vi "Topo & GridSpectr_DriftCorrection_zSpec_v20.vi"(6 "Internal use":string, 7 "Grid param":T2 {"height (m)" format="%#_6p"; "width (m)" format="%#_6p"; "center Y (m)" format="%#_6p"; "center X (m)" format="%#_6p"}, 8 "Error in (no error)":errorcluster, 9 "Points Y/Index Y":i32, 10 "Points X/Index X":i32, 11 "Method":enum16{"init", "run", "end"}(ring)=enum."end") -> (0 "Error out":errorcluster)   [LabVIEW 2014]
doc: "Example of a measurement VI to be used in the \"Experiments on a Grid\" tool as external VI.\n\nThis example measure the topography and spectroscopy data. The spectroscopy measurements are taken on a subgrid. The data are saved to a sxm and a binary file.\n\n- Nanonis Programming Interface -"
uses:
  <userlib>/Nanonis Prog Interface V5/Nanonis Prog Interface.lvlib
panel:
  out "output cluster":T1
  in  "PLL ON/OFF":bool=TRUE
  in  "Spectroscopy":u16(ring) items=["Bias", "zSpec"]
  in  "autoStop":bool
  in  "trigger 2 >Hz":sgl format="%#_6p"
  in  "trigger1 < Hz":sgl format="%#_6p"
  out "zFile":refnum<file>
  out "last z adjustment":sgl=-8.2707174e-12 format="%#_6p"
  in  "during Spec Bias (V)":sgl=-0.1 format="%#_5p"
  in  "type":u16(ring)=1 items=["Line", "Grid"]
  in  "readjust setpoint every":i32=1
  in  "Correct Drift":bool=TRUE
  in  "Email when finished":string="cornelius.krull@monash.edu,Dhaneesh.Gopalakrishnan@monash.edu,marina.castelli@monash.edu"
  in  "STS z offset":dbl=2e-10 format="%#_6p"
  out "ETA":timestamp=timestamp(3575267058.899443 s since 1904-01-01)
  out "remaining":dbl format="%<%H:%M:%S>t"
  out "Progress":u8(slide)=100 scale=0.0..100.0 scale format="%#.1g"
  out "total Points":i32=2500
  in  "preSTS delay [ms]":u32=500
  in  "ref Bias":dbl=-0.1 format="%#_6p"
  in  "Imaging Bias":dbl=0.02 format="%#_6p"
  in  "max applied Drift Correction":i32=20 min=1 max=100 step=1 format="%.0p"
  in  "Correlate":u16(ring) items=["first Frame", "successive Frames"]
  out "Topo Images taken":i32=50
  in  "Increment":i32=8
  in  "Threshold":i32=2 min=1 step=1
  in  "tip Speed (m/s)":sgl=2e-09 format="%.2p"
  out "X drift":i32=1
  out "Y drift":i32
  out "Last Drift detected":i32=1
  in  "MaxImagesBack":i32=2
  in  "Channel index (0-23)":u8(ring) items=["Current"=0, "Z (m)"=14]
  in  "File name":string="symmetric_node_zOff=200p"
  in  "ref Current":dbl=7e-11 format="%#_6p"
  in  "Imaging Current":dbl=1e-11 format="%#_6p"
  in  "zdrift \nDuration (s)":dbl
  in  "Correct z drift":bool
  out "Status":string="finishing"
  in  "Drift correction Pixels":i32=256 caption="Topo Pixels"
  out "Y Offset":dbl=-4.101562475072873e-10 format="%#_6p"
  out "X Offset":dbl=4.687499971511855e-10 format="%#_6p"
  out "Points taken":dbl=2500.0
  in  "Drift Correction every":i32=80
  # "z Spectroscopy"
  # "GRID points"
  # "Increase this if no Drift was detected for \na certain number of images"
  # "%"
  # "time (HH:MM:SS)"
  # "images back"
  # "% of image size"
  # "RUN smart tilt before starting the GRID\nImg Angle = 0  CHECK CUTOFF\nmove tip to reference point for tip height"
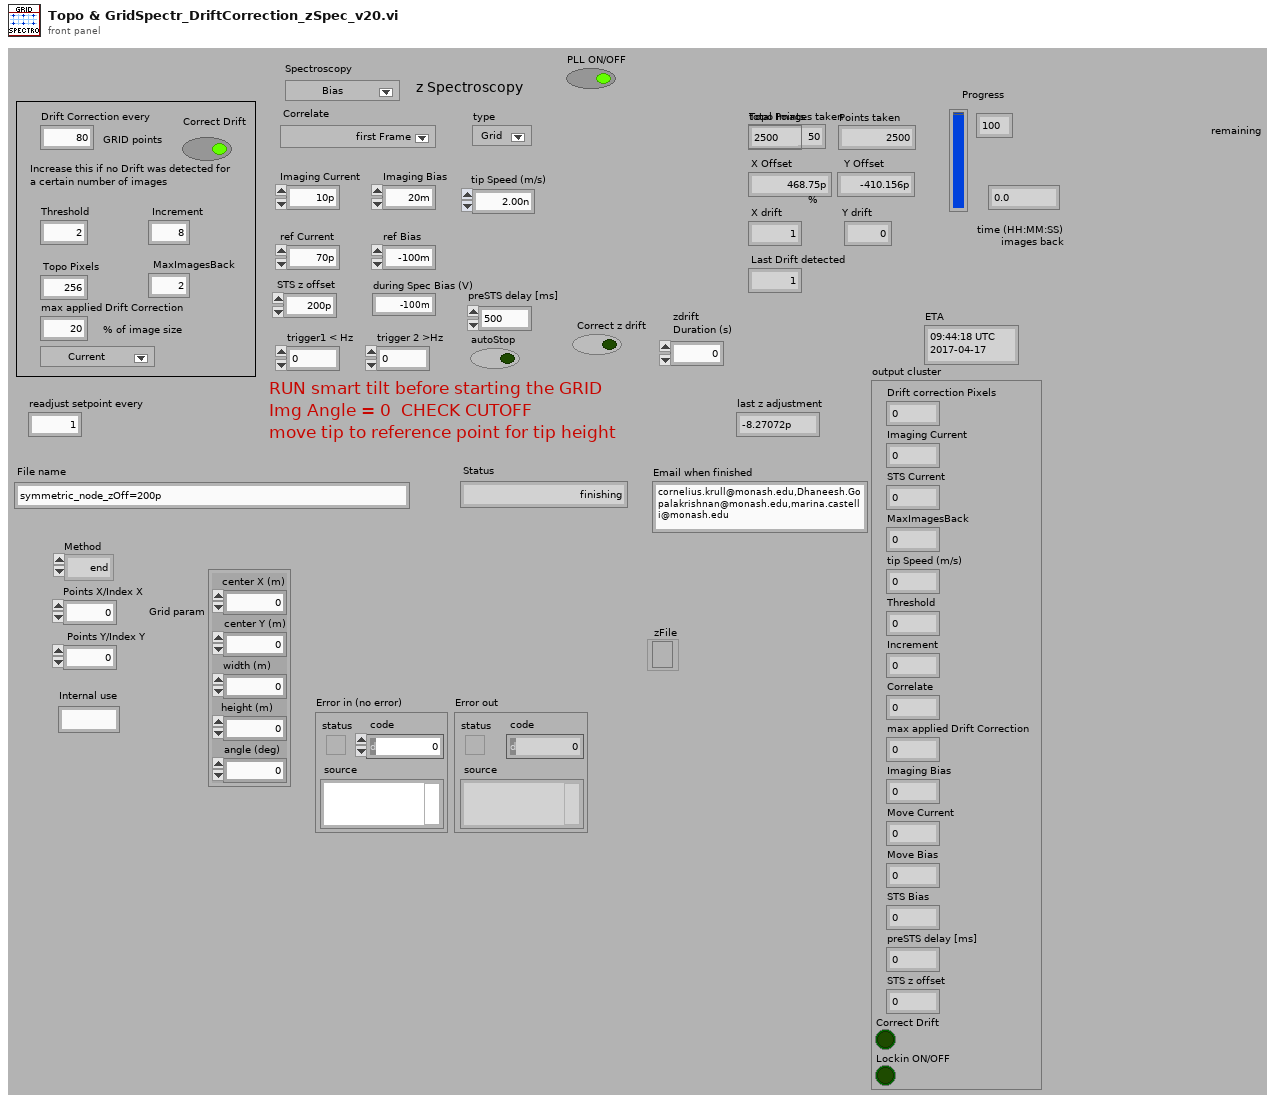
[diagram p1: front panel]
types:
  T1 = cluster{"Drift correction Pixels":i32, "Imaging Current":dbl, "STS Current":dbl, "MaxImagesBack":i32, "tip Speed (m/s)":sgl, "Threshold":i32, "Increment":i32, "Correlate":u16, "max applied Drift Correction":i32, "Imaging Bias":dbl, "Move Current":dbl, "Move Bias":dbl, "STS Bias":dbl, "preSTS delay [ms]":u32, "STS z offset":dbl, "Correct Drift":bool, "Lockin ON/OFF":bool}
  T2 = cluster{"center X (m)":sgl, "center Y (m)":sgl, "width (m)":sgl, "height (m)":sgl, "angle (deg)":sgl}
  T3 = cluster{"Z averaging time (s)":sgl, "Z offset (m)":sgl, "Initial settling time (s)":sgl}
  T4 = cluster{"center X":sgl, "center Y":sgl, "angle":sgl, "width":sgl, "height":sgl, "# pixels":i32, "# lines":i32}
  T5 = cluster{"Name":string, "Calibration":sgl, "Offset":sgl, "Channel index":i32}[]
  T6 = cluster{"up/down":bool, "time/line":sgl, "start time":timestamp, "end time":timestamp}
  T7 = cluster{"Max. slew rate (V/s)":sgl, "Settling time (s)":sgl, "Integration time (s)":sgl}
  T8 = cluster{"End settling time (s)":sgl, "Z control time (s)":sgl}
  T9 = cluster{"Z averaging time (s)":sgl, "Initial settling time (s)":sgl}
  T10 = cluster{"Max. slew rate (m/s)":sgl, "Settling time (s)":sgl, "Integration time (s)":sgl}
  T11 = cluster{"Points X/Index X":i32, "Points Y/Index Y":i32}
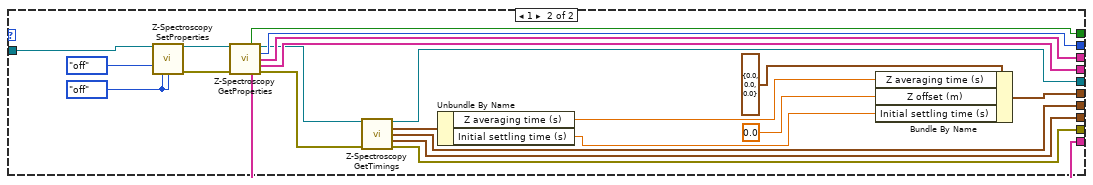
[diagram p2: hidden frame]
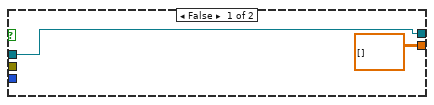
[diagram p3: hidden frame]
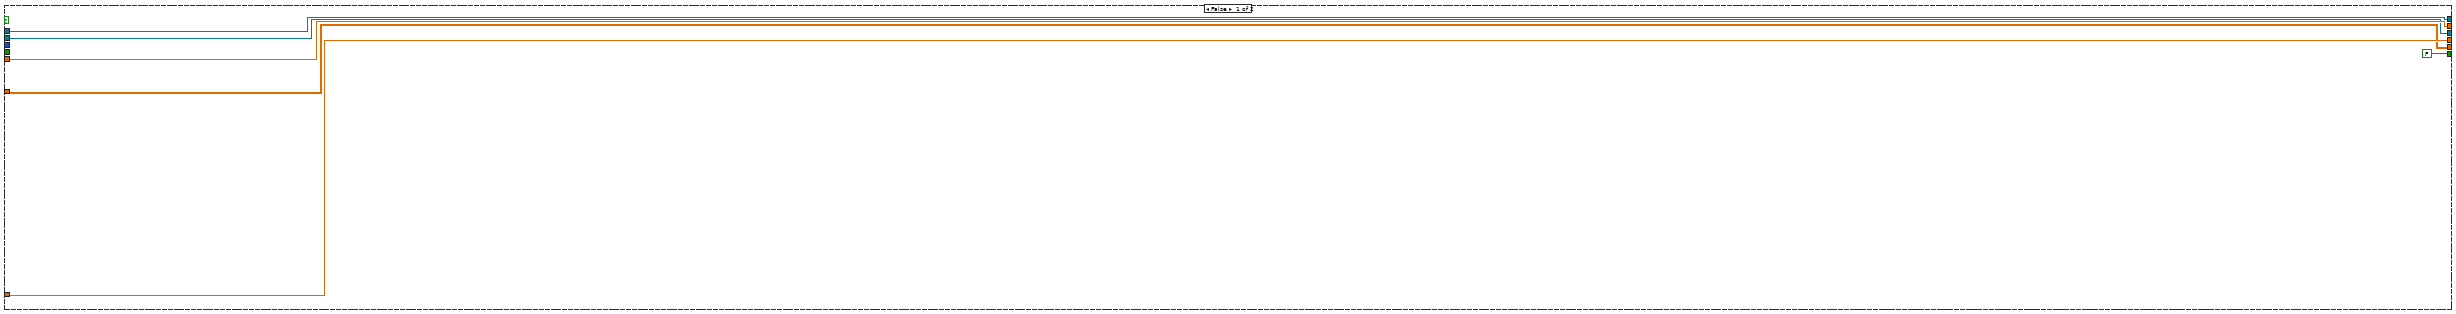
[diagram p9: hidden frame]
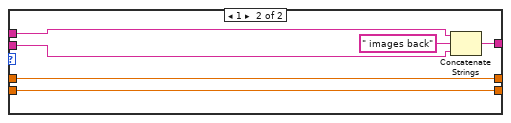
[diagram p10: hidden frame]
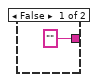
[diagram p12: hidden frame]
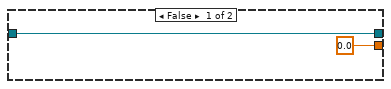
[diagram p13: hidden frame]
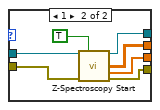
[diagram p15: hidden frame]
diagram:
  n1 = while {
    shift-right: [w22] -> _
    shift-left: _ -> [w38]
    shift-right: [w34] -> _
    shift-left: _ -> [w33]
    shift-right: [w31] -> _
    shift-left: _ -> [w32]
    shift-right: [w30] -> _
    shift-left: _ -> [w29]
    shift-right: [w28] -> _
    shift-left: _ -> [w27]
    shift-right: [w26] -> _
    shift-left: _ -> [w25]
    shift-right: [w24] -> _
    shift-left: _ -> [w23]
    shift-right: [w21] -> _
    shift-left: _ -> [w20]
    shift-right: [w19] -> _
    shift-left: _ -> [w18]
    shift-right: [w17] -> _
    shift-left: _ -> [w10]
    shift-right: [w16] -> _
    shift-left: _ -> [w9]
    shift-right: [w15] -> _
    shift-left: _ -> [w12]
    shift-right: [w14] -> _
    shift-left: _ -> [w11]
    shift-right: [w7] -> _
    shift-left: _ -> [w6]
    stop <- TRUE stop-if-true
    n2 = case shown="\"init\", Default" "Method" {
      tunnel: [w55 w259 _] -> w22
      tunnel: w38 -> [_ w259 w496]
      tunnel: "Error in (no error)" -> [w114 w252 w524]
      tunnel: [w98 w258 w464] -> w36
      tunnel: "Points X/Index X" -> [w54 w253 _]
      tunnel: "Points Y/Index Y" -> [w53 w246 _]
      tunnel: [w140 w256 w513] -> w34
      tunnel: w33 -> [_ w257 w513]
      tunnel: w32 -> [_ w255 w506]
      tunnel: [w132 w254 _] -> w31
      tunnel: [w130 w196 w536] -> w30
      tunnel: w29 -> [_ w196 w536]
      tunnel: [w89 w239 w475] -> w28
      tunnel: w27 -> [_ w223 w500]
      tunnel: ["Grid param" w249 _] -> w26
      tunnel: w25 -> [_ w249 w523]
      tunnel: [w112 w214 _] -> w24
      tunnel: w23 -> [_ w214 w531]
      tunnel: [w53 w247 w514] -> w21
      tunnel: w20 -> [_ w247 w514]
      tunnel: [w54 w248 w515] -> w19
      tunnel: w18 -> [_ w248 w515]
      tunnel: [w123 w229 w512] -> w17
      tunnel: [w123 w234 w510] -> w16
      tunnel: [w108 w228 w507] -> w15
      tunnel: [0 w212 w511] -> w14
      tunnel: w11 -> [_ w198 w511]
      tunnel: "Drift Correction every" -> [_ w242 _]
      tunnel: w12 -> [_ w233 w507]
      tunnel: w10 -> [_ w240 w512]
      tunnel: w9 -> [_ w226 w510]
      tunnel: "Drift correction Pixels" -> [w107 _ _]
      tunnel: [w86 w231 _] -> w7
      tunnel: w6 -> [_ w232 w508]
      tunnel: "Correct z drift" -> [_ w230 _]
      tunnel: "Channel index (0-23)" -> [w69 w227 _]
      tunnel: "MaxImagesBack" -> [w106 _ _]
      tunnel: "Correlate" -> [w94 _ _]
      frame "init", Default {
        w57 = 0.0 ("Move Current")
        w123 = 0.0
        # "- Get bias spectroscopy parameters\n- Open binary file for spectr. data"
        # "initialize Z buffer"
        # "Get index of Z in Signal list"
        n3 = case shown="0, Default" w94 {
          frame 0, Default {
            n4 = local write "MaxImagesBack"(2 ("StepsBack")) -> ()
          }
          frame 1 {
          }
        }
        n5 = call <userlib>:"Prog Interface - OpenAppRef.vi"("Error in (no error)"=w114) -> ("Error out"=w65:errorcluster, "Application reference"=w66:refnum<vi>)  [unwired: 5 in]
        n6 = local write "Status"("init" ("Status")) -> ()
        n7 = call "Set_reference_Point (SubVI).vi"("error in (no error)"=w65, "Application in"=w66) -> ("error out"=w45:errorcluster, "Application out"=w61:refnum<vi>)  [unwired: 8 in]
        n8 = local write "Topo Images taken"(0 ("Images taken")) -> ()
        n9 = call "Get_GridParams (SubVI).vi"("error in (no error)"=w45, 10:"type", "Application in"=w61) -> ("error out"=w44:errorcluster, "total Points"=→"total Points":i32, "Application out"=w50:refnum<vi>)  [unwired: 5 in, 1 out]
        n10 = local write "Last Drift detected"(0 ("Last Drift detected")) -> ()
        n11 = call <userlib>:"Get Session Path.vi"("error in (no error)"=w44, "Application ref in"=w50) -> ("error out"=w113:errorcluster, "Session path"=w100:path, "Application ref out"=w96:refnum<vi>)  [unwired: 7 in]
        n12 = local read "Spectroscopy"() -> (w51:u16)
        n13 = Get Date/Time In Seconds() -> (seconds since 1Jan1904=w112:timestamp)
        n14 = case shown="0, Default" w51 {
          tunnel: [w142 w177] -> w136
          tunnel: [w145 w176] -> w134
          tunnel: [w149 w163] -> w133
          tunnel: [w144 w175] -> w129
          tunnel: [w143 w174] -> w127
          tunnel: [w146 w173] -> w126
          tunnel: w96 -> [w151 w166]
          tunnel: [w148 w171] -> w64
          tunnel: [w147 w170] -> w63
          tunnel: [w141 w156] -> w49
          tunnel: [w150 w169] -> w52
          frame 0, Default {
            n15 = call <userlib>:"BiasSpectroscopy SetProperties.vi"("Application ref in"=w151) -> ("Application ref out"=w155:refnum<vi>, "Error out"=w154:errorcluster)  [unwired: 13 in]
            n16 = call <userlib>:"BiasSpectroscopy GetProperties.vi"("Application ref in"=w155, "Error in (no error)"=w154) -> ("Backward sweep"=w142:bool, "Application ref out"=w153:refnum<vi>, "Number of points"=w143:i32, "Channels"=w146:string[], "Parameters"=w145:string[], "Fixed parameters"=w144:string[], "Error out"=w152:errorcluster)  [unwired: 5 in, 2 out]
            n17 = call <userlib>:"BiasSpectroscopy GetTimings.vi"("Application ref in"=w153, "Error in (no error)"=w152) -> ("Application ref out"=w150:refnum<vi>, "Initialization"=w141:T3, "Sweep Timing"=w147:T7, "End of Sweep"=w148:T8, "Error out"=w149:errorcluster)  [unwired: 9 in]
          }
          frame 1 {
            w168 = enum16{"no change", "on", "off"}."off" ("Save dialog")
            n18 = call <userlib>:"Z-Spectroscopy SetProperties.vi"("Application ref in"=w166, "Autosave"=enum16{"no change", "on", "off"}."off" ("Autosave (no change)"), "Save dialog"=w168, "Save all sweeps (no change)"=w168) -> ("Application ref out"=w165:refnum<vi>, "error out"=w164:errorcluster)  [unwired: 10 in]
            n19 = call <userlib>:"Z-Spectroscopy GetProperties.vi"("Application ref in"=w165, "error in (no error)"=w164) -> ("Backward sweep"=w177:bool, "Application ref out"=w172:refnum<vi>, "Number of points"=w174:i32, "Channels"=w173:string[], "Parameters"=w176:string[], "Fixed parameters"=w175:string[], "error out"=w162:errorcluster)  [unwired: 6 in, 1 out]
            n20 = call <userlib>:"Z-Spectroscopy GetTimings.vi"("Application ref in"=w172, "Error in (no error)"=w162) -> ("Application ref out"=w169:refnum<vi>, "Initialization"=w157:T9, "Sweep Timing"=w170:T10, "End of Sweep"=w171:T8, "Error out"=w163:errorcluster)  [unwired: 9 in]
            n21 = Unbundle By Name(w157) -> ("Z averaging time (s)"=w159:sgl, "Initial settling time (s)"=w160:sgl)
            n22 = Bundle By Name(cluster=T3 {"Z averaging time (s)"=0.0, "Z offset (m)"=0.0, "Initial settling time (s)"=0.0} ("Initialization"), "Z averaging time (s)"=w159, "Z offset (m)"=sgl 0.0, "Initial settling time (s)"=w160) -> (w156:T3)
          }
        }
        n23 = call "Create Filenames (SubVI).vi"("error in (no error)"=w113, "seconds since 1Jan1904"=w112, "File name"="File name", "Session path"=w100) -> ("error out"=w103:errorcluster, "binFilePath"=w99:path, "topoFilePath"=w55:path, "Drift File out"=w87:refnum<file>, 4:w42, 5:→"zFile")  [unwired: 2 in]
        n24 = local read "max applied Drift Correction"() -> (w75:i32)
        n25 = local read "Drift correction Pixels"() -> (w83:i32)
        n26 = local read "preSTS delay [ms]"() -> (w72:u32)
        n27 = local read "Imaging Current"() -> (w82:dbl)
        n28 = local read "MaxImagesBack"() -> (w79:i32)
        n29 = local read "tip Speed (m/s)"() -> (w80:sgl)
        n30 = local read "Imaging Bias"() -> (w74:dbl)
        n31 = local read "Correct Drift"() -> (w70:bool)
        n32 = local read "STS z offset"() -> (w71:dbl)
        n33 = local read "ref Current"() -> (w81:dbl)
        n34 = local read "Increment"() -> (w77:i32)
        n35 = local read "Threshold"() -> (w78:i32)
        n36 = local read "Correlate"() -> (w76:u16)
        n37 = local read "ref Bias"() -> (w73:dbl)
        n38 = Bundle By Name(cluster=T1 {"Drift correction Pixels"=256, "Imaging Current"=5e-11, "STS Current"=1e-10, "MaxImagesBack"=2, "tip Speed (m/s)"=1e-08, "Threshold"=2, "Increment"=64, "Correlate"=0, "max applied Drift Correction"=20, "Imaging Bias"=-0.02, "Move Current"=1.5e-11, "Move Bias"=-0.02, "STS Bias"=0.1, "preSTS delay [ms]"=1000, "STS z offset"=-1.7e-10, "Correct Drift"=TRUE, "Lockin ON/OFF"=TRUE} ("Drift Correction"), "Drift correction Pixels"=w83, "Imaging Current"=w82, "STS Current"=w81, "MaxImagesBack"=w79, "tip Speed (m/s)"=w80, "Threshold"=w78, "Increment"=w77, "Correlate"=w76, "max applied Drift Correction"=w75, "Imaging Bias"=w74, "Move Current"=w57, "Move Bias"=w57, "STS Bias"=w73, "preSTS delay [ms]"=w72, "STS z offset"=w71, "Correct Drift"=w70, "Lockin ON/OFF"=FALSE) -> (→"output cluster":T1)
        n39 = Bundle("Points X/Index X"=w54, "Points Y/Index Y"=w53) -> (w135:T11)  [unwired: 1 in]
        n40 = call "DriftFileHeaderV2 (SubVI).vi"("Byte Stream File in"=w87, "End of Sweep"=w64, "Application ref in"=w52, "Sweep Timing"=w63, "Initialization"=w49) -> ("Byte Stream File out"=w86:refnum<file>, "Application ref out"=w85:refnum<vi>)  [unwired: 8 in, 1 out]
        n41 = call <userlib>:"Create Header for BinaryFile.vi"("Grid points"=w135, "Grid param"="Grid param", "Fixed parameters"=w129, "Backward sweep"=w136, "Sweep signal"="Bias (V)" ("Sweep Signal"), "Parameters"=w134, "Channels"=w126, "Points per sweep"=w127) -> ("Header (fixed attributes)"=w138:string[][])  [unwired: 3 in]
        n42 = call <userlib>:"Write Header to BinaryFile [ with Save dialog].vi"("Fixed Attributes"=w138, "Show Dialog? (T)"=FALSE, "Filename"=w99) -> ("Error out"=w104:errorcluster, "File ref"=w132:refnum<file>)  [unwired: 5 in, 2 out]
        n43 = local read "Imaging Bias"() -> (w91:dbl)
        n44 = Merge Errors(w104, w103) -> (w105:errorcluster)
        n45 = Merge Errors(w133, w105) -> (w98:errorcluster)
        n46 = call "SafeBiasSet.vi"("Application ref in"=w85, "Bias (V)"=w91) -> ("Application ref out"=w48:refnum<vi>)  [unwired: 7 in, 1 out]
        n47 = call <userlib>:"Set Session Path.vi"("error in (no error)"=w98, "Session Folder"=w42, "Application ref in"=w48) -> ("error out"=w97:errorcluster, "Application ref out"=w47:refnum<vi>)  [unwired: 7 in]
        n48 = local read "Imaging Current"() -> (w90:dbl)
        n49 = call <userlib>:"Z-Ctrl Setpoint Set.vi"("error in (no error)"=w97, "Z Controller setpoint"=w90, "Application ref in"=w47) -> ("error out"=w115:errorcluster, "Application ref out"=w116:refnum<vi>)  [unwired: 7 in]
        n50 = call <userlib>:"Signal Names Get.vi"("error in (no error)"=w115, "Application ref in"=w116) -> ("error out"=w68:errorcluster, "Signals Names"=w128:string[], "Application ref out"=w119:refnum<vi>)  [unwired: 5 in]
        n51 = Search 1D Array(1D array=w128, element="Z (m)") -> (index of element=w130:i32)  [unwired: 1 in]
        n52 = call <userlib>:"Scan SetProperties.vi"("Application ref in"=w119, "Continuous scan"=enum16{"No change", "On", "Off"}."Off") -> ("Application ref out"=w121:refnum<vi>, "Error out"=w120:errorcluster)  [unwired: 12 in]
        n53 = call <userlib>:"ScanBuffer Set.vi"("Application ref in"=w121, "Pixels"=w107, "Lines"=w107, "error in (no error)"=w120) -> ("Application ref out"=w92:refnum<vi>)  [unwired: 10 in, 1 out]
        n54 = call <userlib>:"FolMe Speed Set.vi"("Speed Setting (Custom)"=enum32{"Scan speed", "Custom speed"}."Custom speed", "Speed (m/s)"="tip Speed (m/s)", "Application ref in"=w92) -> ("Application ref out"=w60:refnum<vi>)  [unwired: 5 in, 1 out]
        n55 = local read "Correct Drift"() -> (w58:bool)
        n56 = case shown="True" w58 {
          tunnel: w69 -> [_ w189]
          tunnel: w68 -> [_ w188]
          tunnel: [dbl[][] [] ("Array") w187] -> w67
          tunnel: w60 -> [w179 w185]
          tunnel: [w179 w181] -> w56
          frame False {
          }
          frame True {
            n57 = call "PLL_On_Off (SubVI).vi"("Output ON/OFF (F=OFF)"=FALSE, "Application in"=w185) -> ("Application out"=w184:refnum<vi>)  [unwired: 8 in, 1 out]
            n58 = local read "PLL ON/OFF"() -> (w180:bool)
            n59 = call "Scan_normailze(SubVI).vi"("error in (no error)"=w188, "Channel index (0-23)"=w189, "Normalization"=FALSE ("Boolean"), "Application in"=w184) -> ("Array"=w187:dbl[][], "Application out"=w182:refnum<vi>)  [unwired: 5 in, 1 out]
            n60 = call "PLL_On_Off (SubVI).vi"("Output ON/OFF (F=OFF)"=w180, "Application in"=w182) -> ("Application out"=w181:refnum<vi>)  [unwired: 8 in, 1 out]
          }
        }
        n61 = Initialize Array(0.0 ("element"), w106, w107, w107) -> (w109:dbl[][][])
        n62 = for {
          N: w106 -> [_]
          tunnel: w67 -> [w193]
          shift-right: [w192] -> w108
          shift-left: w109 -> [w194]
          i -> [w191]
          n63 = Replace Array Subset(array=w194, new element=w193, index (dim 0)=w191) -> (w192:dbl[][][])  [unwired: 2 in]
        }
        n64 = call <userlib>:"BiasSpectroscopy SetProperties.vi"("Application ref in"=w56, "Z-Controller hold (no change)"=enum16{"no change", "on", "off"}."off") -> ("Application ref out"=w89:refnum<vi>)  [unwired: 12 in, 1 out]
        n65 = Initialize Array(sgl nan ("element"), w53, w54) -> (w140:sgl[][])
      }
      frame "run" {
        # "shift tip position"
        # "Get Z position"
        # "- get Z position for topography and store it to Z buffer\n- if x,y indices are a multiple of the spacings, take spectroscopy curve and write data to binary file\ndo drift correction if number of STS position was reached"
        n66 = Quotient & Remainder(x=w198, y=w242) -> (x-y*floor(x/y)=w243:i32)  [unwired: 1 out]
        n67 = Equal To 0?(x=w243) -> (x = 0?=w241:bool)
        n68 = Not Equal To 0?(x=w198) -> (x != 0?=w224:bool)
        n69 = local read "Correct Drift"() -> (w206:bool)
        n70 = Compound Arithmetic op=AND(w224, w241, w206) -> (w225:bool)
        n71 = call <userlib>:"XY-Pos Get.vi"("Wait for newest data (F=False)"=TRUE, "Application ref in"=w223) -> ("Y (m)"=w219:sgl, "X (m)"=w220:sgl, "Application ref out"=w222:refnum<vi>)  [unwired: 5 in, 1 out]
        n72 = case shown="True" w225 {
          tunnel: w222 -> [w320 w332]
          tunnel: [w320 w377] -> w203
          tunnel: w233 -> [w317 w373]
          tunnel: [w319 w375] -> w229
          tunnel: [w318 w374] -> w234
          tunnel: w240 -> [w319 w356]
          tunnel: w226 -> [w318 w354]
          tunnel: [w317 w369] -> w228
          tunnel: w232 -> [w316 w380]
          tunnel: [w316 w379] -> w231
          tunnel: w230 -> [_ w376]
          tunnel: w227 -> [_ w360]
          tunnel: [FALSE TRUE] -> w200
          frame False {
          }
          frame True {
            # "Drift correction \ncompare to the reference image with the previous image \ndx and dy will be applied to the grid coord, \nand the imaging frame will be shifted"
            n73 = Greater Or Equal To 0?(x=w360) -> (x >= 0?=w359:bool)
            n74 = case shown="True" w359 {
              frame False {
              }
              frame True {
                n75 = local read "Topo Images taken"() -> (w395:i32)
                n76 = Increment(x=w395) -> (x+1=w394:i32)
                n77 = local write "Topo Images taken"(w394) -> ()
              }
            }
            n78 = local read "Imaging Bias"() -> (w339:dbl)
            n79 = call "move2mark (SubVI).vi"("Application in"=w332) -> ("Application out"=w331:refnum<vi>)  [unwired: 10 in]
            n80 = local read "Imaging Current"() -> (w338:dbl)
            n81 = local write "Status"("Drift Correction" ("Status")) -> ()
            n82 = call "SafeBiasSet.vi"("Application ref in"=w331, "Bias (V)"=w339) -> ("Application ref out"=w340:refnum<vi>)  [unwired: 7 in, 1 out]
            n83 = call <userlib>:"Z-Ctrl Setpoint Set.vi"("Z Controller setpoint"=w338, "Application ref in"=w340) -> ("Application ref out"=w330:refnum<vi>)  [unwired: 8 in, 1 out]
            n84 = call <userlib>:"Ctrl-on_off Set.vi"("Z Controller ON/OFF"=TRUE, "Application ref in"=w330) -> ("Application ref out"=w328:refnum<vi>)  [unwired: 8 in, 1 out]
            n85 = call "PLL_On_Off (SubVI).vi"("Output ON/OFF (F=OFF)"=FALSE, "Application in"=w328) -> ("Application out"=w327:refnum<vi>)  [unwired: 8 in, 1 out]
            n86 = local read "Drift correction Pixels"() -> (w348:i32)
            n87 = local read "Last Drift detected"() -> (w351:i32)
            n88 = call "Scan_normailze(SubVI).vi"("Channel index (0-23)"=w360, "Normalization"=FALSE ("Boolean"), "Application in"=w327) -> ("Array"=w370:dbl[][], "Application out"=w325:refnum<vi>)  [unwired: 6 in, 1 out]
            n89 = local read "Correlate"() -> (w357:u16)
            n90 = Divide(x="max applied Drift Correction", y=100) -> (x/y=w347:dbl)
            n91 = Multiply(x=w347, y=w348) -> (x*y=w349:dbl)
            n92 = call "PLL_On_Off (SubVI).vi"("Output ON/OFF (F=OFF)"="PLL ON/OFF", "Application in"=w325) -> ("Application out"=w323:refnum<vi>)  [unwired: 8 in, 1 out]
            n93 = call "CorrelImages (SubVI)v2.vi"("last drift detected"=w351, "Correlate"=w357, "Ref Array"=w373, "New Image"=w370) -> ("Y drift"=w345:i32, "X drift"=w342:i32, "Ref Array out"=w369:dbl[][][], "Queue Steps"=w358:i32)  [unwired: 4 in]
            "X drift" <- w342
            "Y drift" <- w345
            "Last Drift detected" <- w358
            n94 = local read "Topo Images taken"() -> (w362:i32)
            n95 = To Long Integer(number=w349) -> (32bit integer=w341:i32)
            n96 = Greater Or Equal?(x=w358, y="Threshold") -> (x >= y?=w364:bool)
            n97 = Greater?(x=w362, y="Threshold") -> (0:w361:bool)
            n98 = call "AbsLimit (SubVI).vi"("in"=w342, "Abslimt"=w341) -> ("Numeric out"=w344:i32)  [unwired: 9 in]
            n99 = call "AbsLimit (SubVI).vi"("in"=w345, "Abslimt"=w341) -> ("Numeric out"=w343:i32)  [unwired: 9 in]
            n100 = And(x=w364, y=w361) -> (x .and. y?=w363:bool)
            n101 = case shown="True" w363 {
              tunnel: ["" w399] -> w365
              frame False {
              }
              frame True {
                n102 = local write "Last Drift detected"(0 ("Last Drift detected")) -> ()
                n103 = local read "Drift Correction every"() -> (w398:i32)
                n104 = Add(x=w398, y="Increment") -> (x+y=w402:i32)
                n105 = local write "Drift Correction every"(w402) -> ()
                n106 = Number To Decimal String(number=w402) -> (decimal integer string=w401:string)  [unwired: 1 in]
                n107 = Concatenate Strings(" Increased DC to every " ("string"), w401) -> (w399:string)
              }
            }
            n108 = local read "Drift correction Pixels"() -> (w367:i32)
            n109 = call "drift_pixel2m (SubVI).vi"("Application in"=w323, "X drift"=w344, "Y drift"=w343, "Drift correction Pixels"=w367) -> ("Application out"=w366:refnum<vi>, "x drift"=w336:sgl, "y drift"=w335:sgl)  [unwired: 2 in, 1 out]
            n110 = call "ShiftFrame (SubVI).vi"("Y shift"=w335, "X shift"=w336, "Application in"=w366) -> ("Application out"=w368:refnum<vi>)  [unwired: 8 in]
            n111 = local read "type"() -> (w322:u16)
            n112 = call "MoveGrid.vi"("type"=w322, "y"=w335, "x"=w336, "Application ref in"=w368) -> ("Application ref out"=w334:refnum<vi>)  [unwired: 6 in, 1 out]
            n113 = call "shift marks (SubVI).vi"("y"=w335, "x"=w336, "Application in"=w334) -> ("Application out"=w333:refnum<vi>)  [unwired: 7 in, 1 out]
            n114 = case shown="True" w376 {
              tunnel: [0.0 ("z drift") w409] -> w378
              tunnel: w333 -> [w404 w408]
              tunnel: [w404 w407] -> w377
              frame False {
              }
              frame True {
                n115 = call "Zdrift_subVi.vi"("Duration"="zdrift \nDuration (s)", "Application in"=w408) -> ("z drift"=w409:dbl, "Application out"=w407:refnum<vi>)  [unwired: 7 in, 1 out]
              }
            }
            n116 = Number To Decimal String(number=w358) -> (decimal integer string=w372:string)  [unwired: 1 in]
            n117 = case shown="0, Default" w357 {
              tunnel: w372 -> [w382 w393]
              tunnel: [w387 w392] -> w371
              tunnel: w365 -> [w385 w390]
              tunnel: w356 -> [w383 w389]
              tunnel: [w383 w389] -> w355
              tunnel: w354 -> [w384 w388]
              tunnel: [w384 w388] -> w353
              frame 0, Default {
                n118 = Concatenate Strings(w382, "images back , Correlating first frame " ("string"), w385) -> (w387:string)
              }
              frame 1 {
                n119 = Concatenate Strings(w393, " images back" ("string"), w390) -> (w392:string)
              }
            }
            n120 = Add(x=w355, y=w336) -> (x+y=w375:dbl)
            n121 = Add(x=w335, y=w353) -> (x+y=w374:dbl)
            n122 = local write "X Offset"(w375) -> ()
            n123 = call "Drift Data to file (SubVI).vi"("z drift"=w378, "Comment"=w371, "y Drift"=w374, "X drift"=w375, "Byte Stream File in"=w380) -> ("Byte Stream File out"=w379:refnum<file>)  [unwired: 6 in]
            n124 = local write "Y Offset"(w374) -> ()
          }
        }
        n125 = Quotient & Remainder(x=w198, y="readjust setpoint every") -> (x-y*floor(x/y)=w199:i32)  [unwired: 1 out]
        n126 = Equal To 0?(x=w199) -> (x = 0?=w202:bool)
        n127 = Equal To 0?(x=w198) -> (x = 0?=w197:bool)
        n128 = Add(x=w220, y=w229) -> (x+y=w236:dbl)
        n129 = Add(x=w219, y=w234) -> (x+y=w235:dbl)
        n130 = Compound Arithmetic op=OR(w197, w200, w202) -> (w201:bool)
        n131 = case shown="True" w201 {
          tunnel: [w260 w277] -> w204
          tunnel: w203 -> [w260 w293]
          tunnel: w196 -> [_ w279]
          frame False {
          }
          frame True {
            n132 = call "move2mark (SubVI).vi"("Application in"=w293) -> ("Application out"=w282:refnum<vi>)  [unwired: 10 in]
            n133 = local read "ref Bias"() -> (w292:dbl)
            n134 = call <userlib>:"Signal Value Get (Animation period) v2.vi"("Wait for newest data (F=False)"=TRUE, "Signal index (0-79)"=w279, "Application ref in"=w282) -> ("Signal value"=w275:sgl, "Application ref out"=w281:refnum<vi>)  [unwired: 5 in, 1 out]
            n135 = local read "ref Current"() -> (w289:dbl)
            n136 = local write "Status"("adjust setpoint" ("Status")) -> ()
            n137 = call "SafeBiasSet.vi"("Application ref in"=w281, "Bias (V)"=w292) -> ("Application ref out"=w290:refnum<vi>)  [unwired: 7 in, 1 out]
            n138 = flat-sequence {
              tunnel: w290 -> [w298]
              tunnel: [w295] -> w288
              tunnel: w289 -> [w297]
              tunnel: w288 -> [w301]
              tunnel: [w301] -> w287
              tunnel: "preSTS delay [ms]" -> [w299]
              tunnel: w287 -> [w306]
              tunnel: [w303] -> w291
              tunnel: [w304] -> w285
              tunnel: w291 -> [w310]
              tunnel: "preSTS delay [ms]" -> [w309]
              tunnel: w285 -> [_]
              tunnel: [w310] -> w283
              tunnel: [w312] -> w278
              tunnel: w283 -> [w313]
              frame #0 {
                n139 = call <userlib>:"Z-Ctrl Setpoint Set.vi"("Z Controller setpoint"=w297, "Application ref in"=w298) -> ("Application ref out"=w296:refnum<vi>)  [unwired: 8 in, 1 out]
                n140 = call <userlib>:"Ctrl-on_off Set.vi"("Z Controller ON/OFF"=TRUE, "Application ref in"=w296) -> ("Application ref out"=w295:refnum<vi>)  [unwired: 8 in, 1 out]
              }
              frame #1 {
                n141 = Greater Than 0?(x=w299) -> (x > 0?=w300:bool)
                n142 = case shown="True" w300 {
                  tunnel: w299 -> [_ w302]
                  frame False {
                  }
                  frame True {
                    n143 = Wait (ms)(milliseconds to wait=w302) -> ()  [unwired: 1 out]
                  }
                }
              }
              frame #2 {
                n144 = local read "STS z offset"() -> (w304:dbl)
                n145 = call <userlib>:"TipLift Set.vi"("TipLift (m)"=w304, "Application ref in"=w306) -> ("Application ref out"=w305:refnum<vi>)  [unwired: 8 in, 1 out]
                n146 = call <userlib>:"Ctrl-on_off Set.vi"("Z Controller ON/OFF"=FALSE, "Application ref in"=w305) -> ("Application ref out"=w303:refnum<vi>)  [unwired: 8 in, 1 out]
              }
              frame #3 {
                n147 = Greater Than 0?(x=w309) -> (x > 0?=w308:bool)
                n148 = case shown="True" w308 {
                  tunnel: w309 -> [_ w311]
                  frame False {
                  }
                  frame True {
                    n149 = Wait (ms)(milliseconds to wait=w311) -> ()  [unwired: 1 out]
                  }
                }
              }
              frame #4 {
                n150 = call "SafeBiasSet.vi"("Application ref in"=w313, "Bias (V)"="during Spec Bias (V)") -> ("Application ref out"=w312:refnum<vi>)  [unwired: 7 in, 1 out]
              }
            }
            n151 = Get Date/Time In Seconds() -> (seconds since 1Jan1904=w266:timestamp)
            n152 = call <userlib>:"Signal Value Get (Animation period) v2.vi"("Wait for newest data (F=False)"=TRUE, "Signal index (0-79)"=w279, "Application ref in"=w278) -> ("Signal value"=w274:sgl, "Application ref out"=w277:refnum<vi>)  [unwired: 5 in, 1 out]
            n153 = Get Date/Time String(date format (0)=enum16{"short", "long", "abbreviated"}."short", seconds (now)=w266, want seconds? (F)=TRUE) -> (date string=w270:string, time string=w269:string)
            n154 = Subtract(x=w275, y=w274) -> (x-y=w272:sgl)
            "last z adjustment" <- w272
            n155 = Concatenate Strings(w270, w269, "," ("string")) -> (w268:string)
            n156 = Format Into String(format string="%#g", initial string=w268, w272) -> (resulting string=w263:string)  [unwired: 1 in, 1 out]
            n157 = Concatenate Strings(w263, "\r\n") -> (w262:string)
            n158 = local read "zFile"() -> (w273:refnum<file>)
            n159 = Write to Text File(file (use dialog)=w273, text=w262) -> ()  [unwired: 2 in, 3 out]
          }
        }
        n160 = Subtract(x=w247, y=w246) -> (x-y=w245:i32)
        n161 = call <userlib>:"XY-Pos Set.vi"("Y (m)"=w235, "X (m)"=w236, "Application ref in"=w204) -> ("Application ref out"=w237:refnum<vi>)  [unwired: 5 in, 1 out]
        n162 = Decrement(x=w245) -> (x-1=w244:i32)
        n163 = call <userlib>:"Signal Value Get (Animation period).vi"("error in (no error)"=w252, "Signal index (0-47)"=w196, "Application ref in"=w237) -> ("error out"=w251:errorcluster, "Signal value"=w250:sgl, "Application ref out"=w238:refnum<vi>)  [unwired: 5 in]
        n164 = Replace Array Subset(array=w257, new element=w250, index (row)=w244, index (col)=w253) -> (w256:sgl[][])
        n165 = case shown="True" TRUE {
          tunnel: [w412 w416] -> w258
          tunnel: w255 -> [w413 w436]
          tunnel: [w413 w434] -> w254
          tunnel: w251 -> [w412 w419]
          tunnel: w238 -> [w411 w420]
          tunnel: [w411 w421] -> w239
          tunnel: [w410 w423] -> w212
          tunnel: w198 -> [w410 w424]
          frame False {
            # "Point indices aren't multiple of subgrid spacing\n=> no spectroscopy at this point"
          }
          frame True {
            n166 = local write "Status"("zSpec" ("Status")) -> ()
            n167 = case shown="True" "autoStop" {
              tunnel: w420 -> [_ w456]
              tunnel: w419 -> [w451 w453]
              tunnel: [w451 w452] -> w418
              frame False {
              }
              frame True {
                n168 = call "zSpec_trigger.vi"("Error in (no error)"=w453, "trigger 2"="trigger 2 >Hz", "trigger1"="trigger1 < Hz", "Application ref in"=w456) -> ("Error out"=w452:errorcluster)  [unwired: 5 in, 1 out]
              }
            }
            n169 = case shown="0, Default" "Spectroscopy" {
              tunnel: [w437 w450] -> w433
              tunnel: [w438 w449] -> w432
              tunnel: [w439 w447] -> w426
              tunnel: [w440 w446] -> w421
              tunnel: w420 -> [w442 w445]
              tunnel: w419 -> [w441 w444]
              frame 0, Default {
                n170 = call <userlib>:"BiasSpectroscopy Start.vi"("Application ref in"=w442, "Get data (F)"=TRUE, "Error in (no error)"=w441) -> ("Application ref out"=w440:refnum<vi>, "Data"=w437:sgl[][], "Parameters"=w438:sgl[], "Error out"=w439:errorcluster)  [unwired: 8 in, 1 out]
              }
              frame 1 {
                n171 = call <userlib>:"Z-Spectroscopy Start.vi"("Application ref in"=w445, "Get data (F=False)"=TRUE ("Get Data (F)"), "error in (no error)"=w444) -> ("Application ref out"=w446:refnum<vi>, "Data"=w450:sgl[][], "Parameters"=w449:sgl[], "error out"=w447:errorcluster)  [unwired: 8 in, 1 out]
              }
            }
            n172 = Delete From Array(array=w433, length=1, index (row)=0 ("index")) -> (array with subset deleted=w431:sgl[][])  [unwired: 1 in, 1 out]
            n173 = Write to Binary File(file (use dialog)=w436, data=w432, error in=w426, 5:FALSE ("prepend array or string size? (T)")) -> (refnum out=w435:refnum<file>, error out=w425:errorcluster)  [unwired: 2 in, 1 out]
            n174 = Write to Binary File(file (use dialog)=w435, data=w431, error in=w425, 5:FALSE ("prepend array or string size? (T)")) -> (refnum out=w434:refnum<file>, error out=w417:errorcluster)  [unwired: 2 in, 1 out]
            n175 = Increment(x=w424) -> (x+1=w423:i32)
            n176 = Merge Errors(w418, w417) -> (w416:errorcluster)
          }
        }
        n177 = Get Date/Time In Seconds() -> (seconds since 1Jan1904=w209:timestamp)
        n178 = local read "total Points"() -> (w215:i32)
        n179 = Subtract(x=w209, y=w214) -> (x-y=w213:dbl)
        n180 = Subtract(x=w215, y=w212) -> (x-y=w210:i32)
        n181 = Divide(x=w212, y=w215) -> (x/y=w218:dbl)
        n182 = Divide(x=w213, y=w212) -> (x/y=w211:dbl)
        n183 = Multiply(x=w211, y=w210) -> (x*y=w208:dbl)
        "remaining" <- w208
        n184 = Multiply(x=w218, y=100.0) -> (x*y=→"Progress":dbl)
        n185 = Add(x=w209, y=w208) -> (x+y=→"ETA":timestamp)
      }
      frame "end" {
        n186 = Close File(refnum=w508) -> ()  [unwired: 1 in, 2 out]
        n187 = Unbundle By Name(w523) -> ("center X (m)"=w521:sgl, "center Y (m)"=w520:sgl, "angle (deg)"=w519:sgl, "width (m)"=w518:sgl, "height (m)"=w517:sgl)
        n188 = Bundle(w513, w513) -> (w535:cluster{sgl[][], sgl[][]})  [unwired: 1 in]
        n189 = Strip Path(path=w496) -> (stripped path=w504:path)  [unwired: 1 out]
        n190 = Close File(refnum=w506) -> (path=w505:path)  [unwired: 1 in, 1 out]
        n191 = local write "Status"("finishing" ("Status")) -> ()
        n192 = call "STSGrid.vi"("Binary Spectroscopy File"=w505) -> ()  [unwired: 11 in]
        n193 = Strip Path(path=w504) -> (stripped path=w503:path)  [unwired: 1 out]
        n194 = Build Array(w535) -> (w534:cluster{sgl[][], sgl[][]}[])
        n195 = Bundle By Name(cluster=T4 {"center X"=0.0, "center Y"=0.0, "angle"=0.0, "width"=0.0, "height"=0.0, "# pixels"=0, "# lines"=0} ("Scanfield"), "center X"=w521, "center Y"=w520, "angle"=w519, "width"=w518, "height"=w517, "# lines"=w514, "# pixels"=w515) -> (w516:T4)
        n196 = Path To String(path=w503) -> (string=w461:string)
        n197 = String To Path(string=w461) -> (path=w460:path)
        n198 = Strip Path(path=w496) -> (stripped path=w527:path, name=w526:string)
        n199 = Get Date/Time In Seconds() -> (seconds since 1Jan1904=w492:timestamp)
        n200 = Bundle By Name(cluster=T6 {"up/down"=FALSE, "time/line"=0.0, "start time"=timestamp(0 s since 1904-01-01), "end time"=timestamp(0 s since 1904-01-01)} ("Scan param"), "up/down"=TRUE, "time/line"=sgl nan ("input 7"), "start time"=w531, "end time"=w492) -> (w530:T6)
        n201 = Bundle("stripped path"=w527, "name"=w526) -> (w525:cluster{"stripped path":path, "name":string})  [unwired: 1 in]
        n202 = call <userlib>:"Save sxm File.vi"("Auto file naming? (T)"=FALSE, "Scanfield"=w516, "Scan param"=w530, "error in (no error)"=w524, "Channels data"=w534, "Channels config"=T5 [{"Name"="Z (m)", "Calibration"=1.0, "Offset"=0.0, "Channel index"=0}], "Filename control"=w525) -> ("error out"=w501:errorcluster)  [unwired: 2 in, 2 out]
        n203 = call <userlib>:"Get Session Path.vi"("error in (no error)"=w501, "Application ref in"=w500) -> ("error out"=w497:errorcluster, "Session path"=w499:path, "Application ref out"=w459:refnum<vi>)  [unwired: 7 in]
        n204 = call "SXM.vi"("Path"=w499, "Delete"=FALSE, "error in"=w497) -> ("error out"=w462:errorcluster)  [unwired: 7 in]
        n205 = Format Date/Time String(time format string (%c)=" Finished at %y%m%d - %H%M%S ", seconds (now)=w492) -> (date/time string=w491:string)  [unwired: 1 in]
        n206 = Path To String(path=w496) -> (string=w495:string)
        n207 = call <userlib>:"Set Session Path.vi"("Save settings to previous? (False)"=TRUE, "error in (no error)"=w462, "Session Folder"=w460, "Application ref in"=w459) -> ("error out"=w457:errorcluster, "Application ref out"=w458:refnum<vi>)  [unwired: 6 in]
        n208 = local read "zFile"() -> (w476:refnum<file>)
        n209 = Search and Replace String(input string="Email when finished", search string="@") -> (number of replacements=w487:i32)  [unwired: 6 in, 3 out]
        n210 = Concatenate Strings(w495, "\r\n", w491) -> (w494:string)
        n211 = call <userlib>:"BiasSpectroscopy SetProperties.vi"("Application ref in"=w458, "Z-Controller hold (no change)"=enum16{"no change", "on", "off"}."on") -> ("Application ref out"=w484:refnum<vi>)  [unwired: 12 in, 1 out]
        n212 = Close File(refnum=w476, error in=w457) -> (error out=w472:errorcluster)  [unwired: 1 out]
        n213 = Greater Than 0?(x=w487) -> (x > 0?=w486:bool)
        n214 = case shown="True" w486 {
          tunnel: w472 -> [w537 w542]
          tunnel: w494 -> [_ w540]
          tunnel: "Email when finished" -> [_ w539]
          tunnel: [w537 w538] -> w468
          frame False {
          }
          frame True {
            n215 = call "Send Email"("error in"=w542, "Message"=w540, "Subject"="Grid Finished", "Recipients"=w539) -> ("error out"=w538:errorcluster)  [unwired: 7 in]
          }
        }
        n216 = call <userlib>:"TipLift Set.vi"("TipLift (m)"=sgl 0.0, "Application ref in"=w484) -> ("Application ref out"=w481:refnum<vi>)  [unwired: 8 in, 1 out]
        n217 = call "move2mark (SubVI).vi"("Application in"=w481) -> ("Application out"=w467:refnum<vi>)  [unwired: 10 in]
        n218 = local read "Imaging Current"() -> (w465:dbl)
        n219 = call <userlib>:"Z-Ctrl Setpoint Set.vi"("Z Controller setpoint"=w465, "Application ref in"=w467) -> ("Application ref out"=w466:refnum<vi>)  [unwired: 8 in, 1 out]
        n220 = local read "Imaging Bias"() -> (w477:dbl)
        n221 = call "SafeBiasSet.vi"("Application ref in"=w466, "Bias (V)"=w477, "error in (no error)"=w468) -> ("Application ref out"=w478:refnum<vi>, "Error out"=w471:errorcluster)  [unwired: 6 in]
        n222 = call <userlib>:"Ctrl-on_off Set.vi"("error in (no error)"=w471, "Z Controller ON/OFF"=TRUE, "Application ref in"=w478) -> ("error out"=w470:errorcluster, "Application ref out"=w480:refnum<vi>)  [unwired: 7 in]
        n223 = call <userlib>:"Point Erase.vi"("Application ref in"=w480, "Point index (-1=All points)"=0, "error in (no error)"=w470) -> ("Application ref out"=w474:refnum<vi>, "error out"=w469:errorcluster)  [unwired: 11 in]
        n224 = call "PLL_On_Off (SubVI).vi"("error in (no error)"=w469, "Output ON/OFF (F=OFF)"=FALSE, "Application in"=w474) -> ("error out"=w464:errorcluster, "Application out"=w475:refnum<vi>)  [unwired: 7 in]
      }
    }
    "Error out" <- w36
    "Points taken" <- w11
    "X Offset" <- w10
    "Y Offset" <- w9
  }
